vi "environment_get.vi"(0 "reference":refnum<class "OSA.lvclass">, 3 "read defaultValues":bool, 5 "error in (no error)":errorcluster, 9 "parameter":T1(ring)) -> (8 "update temp":bool, 10 "update pressure":bool, 12 "update humidity":bool, 14 "duplicate reference":refnum<class "OSA.lvclass">, 15 "temp (degree C)":sgl format="%.2f", 16 "rel humidity (%)":sgl, 17 "pressure (hPa)":sgl format="%.2f", 19 "error out":errorcluster)   [LabVIEW 2010, in "OSA.lvclass"]
doc: "Interferometer environment."
uses:
  OSA.lvclass
  FTSLib.dll
panel:
  out "par option":i32 format="%b"
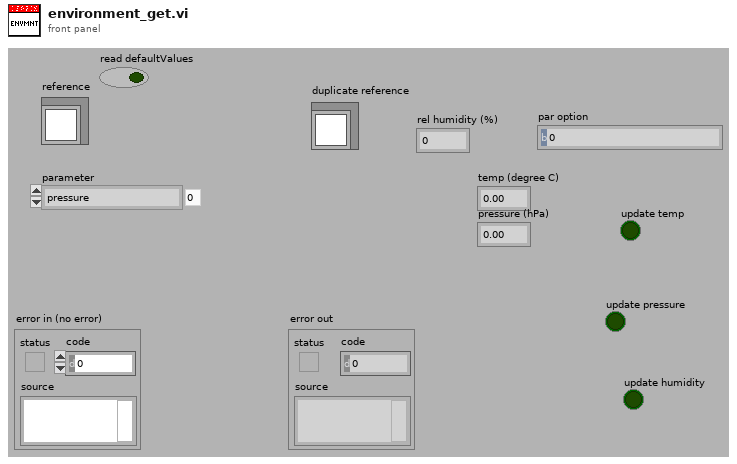
[diagram p1: front panel]
types:
  T1 = enum16{"pressure", "temperature", "humidity", "all"}
  T2 = typedef "OSA.lvclass/ObjectAttributes.ctl" = cluster{"Stop":bool, "dataType":T3, "spectrometerIdx":u16, "buffer size interferogram":i32, "interferogram":cluster{"new":bool, "plot_x_ min":sgl, "plot_x_max":sgl, "plot_y_min":sgl, "plot_y_max":sgl, "Graph Intrfrgrm":T4, "timeStamp":u32, "signal (%)":dbl, "traces":cluster{"idx":u32, "broadBand":bool, "monoChromatic":bool, "peakToPeakSignal":dbl, "peakToPeakPos":dbl}[], "traces idx last":i32, "contrast (%)":dbl}, "spectrum":cluster{"new":bool, "plot_x_min":sgl, "plot_x_max":sgl, "plot_unit_x":T5, "plot_unit_y":T6, "plot_y_min":sgl, "plot_y_max":sgl, "Graph Spectrum":T4, "timeStamp":u32, "X_VAL_OPTIONS":enum16{"MIN_MAX", "ARRAY"}, "traces":cluster{"idx":u32}[], "traces idx last":i32}, "Thorlabs_OSA_64.lvclass:queue_action.ctlqueue ref":refnum<queue>, "action":T7, "plot zoom step":dbl, "buffer semaphore":T8, "acq stopped":bool, "dataType active":T3, "temperature (degr C)":sgl, "pressure (hPa)":sgl, "rel humidity (%)":sgl, "settings":cluster{"resolution":u16, "sensitivity":u16, "Average":bool, "average nr":u32, "apodisation":T9, "acq delay (ms)":u32, "airMesure":T10, "wmtr on":bool, "intfgrm_smooth_width":u16, "intfgrm_smooth_nrOfPasses":u16, "intfgrm_smooth":T11, "phaseCorrection":T12, "zeroFill":u8, "spectr_smooth":T11, "spectr_smooth_width":u16, "spectr_smooth_nrOfPasses":u16, "resolution (/cm)":sgl, "REF wavelength, (nm)":dbl, "gain_idx":u16, "gainAuto":bool, "gain_relative":dbl, "PD sensitivity mode":T13, "PD senseMode implemented":bool, "SensorTemperature implemented":bool, "SensorPressure implemented":bool, "SensorHumidity implemented":bool, "attenuationAuto":bool, "attenuationOnOff":bool, "attenuationAvailable":bool, "offsetAvailable":bool, "offset":i32, "offset max":u16, "contrastAvailable":bool}, "peaks position":sgl[], "peaks width":sgl[], "peaks height":sgl[], "peaks max nr":u32, "peaks latest nr":i32, "peaks new":bool, "power":dbl, "power new":bool, "path":string, "wavelength (WNr)":dbl, "wavelength new":bool, "buffer size spectrum":i32, "status":string, "vi reference":refnum<vi>, "funcPointer":u64, "libraryPointer":u64, "singleAcquisition":bool, "coherenceLength (cm)":dbl, "coherenceLength new":bool, "spectrometer model":string, "spectrometer serial nr":string, "peaks thld left":sgl[], "peaks thld right":sgl[], "coherenceLength error (cm)":dbl, "ADC bits":u16, "peaks position centroid":sgl[], "peaks height centroid":sgl[], "OSA series":T14, "channel index spectrum":u16, "spectrometer rangeLow, (/cm)":dbl, "spectrometer rangeHigh, (/cm)":dbl, "channel index interferogram":u16, "virtualSource":bool, "sweep restart":bool}
  T3 = typedef "OSA.lvclass/acq_dataType.ctl" = enum16{"none", "interferogram", "spectrum"}
  T4 = typedef "OSA.lvclass/graph_intensity.ctl" = refnum<vi>
  T5 = typedef "OSA.lvclass/spectrum_x_unit.ctl" = enum16{"wavenr/cm", "THz", "eV", "nm_air", "nm_vac"}
  T6 = typedef "OSA.lvclass/y_unit.ctl" = enum16{"ADC counts", "dBm pwr absolute", "dBm pwr density", "mW pwr absolute", "mW pwr density"}
  T7 = typedef "OSA.lvclass/queue_action.ctl" = enum16{"none", "stop", "GUI_plotInterferogram", "GUI_plotSpectrum", "GUI_plotInterferogramRescale", "GUI_plotSpectrumRescale", "GUI_plotInterferogramReset", "GUI_plotSpectrumReset", "GUI_plotInterferogramAutoScaleY", "GUI_plotSpectrumAutoScaleY", "GUI_plotInterferogramZoomOut", "GUI_plotSpectrumZoomOut", "GUI_plotInterferogramPane", "GUI_plotSpectrumPane", "GUI_plotInterferogramZoomMouse", "GUI_plotSpectrumZoomMouse", "GUI_spectrumChannelType", "GUI_channel", "ENVIRONMENT temperature", "ENVIRONMENT pressure", "MODE_resolution set", "MODE_resolution get", "MODE_sensitivity set", "MODE_sensitivity get", "MODE_PDTemperature set", "MODE_PDTemperature get", "REBOOT/RESET firmware", "ACQASYNC_acquireSingleSpectrum", "ACQASYNC_continuous start", "ACQASYNC_continuous stop\n", "ACQASYNC_get last interferogram", "ACQASYNC_get last spectrum", "ACQASYNC_get last waveNr", "ACQOPT_interferogram smoothing set", "ACQOPT_interferogram smoothing get", "ACQOPT_spectrum smoothing set", "ACQOPT_spectrum smoothing get", "ACQOPT_apodisation type set", "ACQOPT_apodisation type get", "ACQOPT_phase correction type set", "ACQOPT_phase correction type get", "ACQOPT_acqIntervall_set", "ACQOPT_acqIntervall_get", "ACQOPT_average spectrum set", "ACQOPT_average spectrum get", "ACQOPT_rolling average set", "ACQOPT_rolling average get", "ACQOPT_zero fill factor set", "ACQOPT_zero fill factor get", "ACQOPT_cycle counting set", "ACQOPT_cycle counting get", "ACQOPT_air measure option set", "ACQOPT_air measure option get", "ACQOPT_gainLevel auto get", "ACQOPT_gainLevel auto set", "ACQOPT_gainLevel get", "ACQOPT_gainLevel set", "ACQOPT_offset set", "ACQOPT_attenuator_auto_set", "ACQOPT_attenuator_set", "ACQOPT_getAll", "INSTRUMENT_PROPERTY_range_WaveNr_min", "INSTRUMENT_PROPERTY_range_WaveNr_max", "INSTRUMENT_PROPERTY_reference_wavelength_cm^-1", "INSTRUMENT_PROPERTY_samplesPerRefPeriod", "INSTRUMENT_PROPERTY_resolution_waveNrPercm", "INSTRUMENT_PROPERTY_availableGainLevels", "INSTRUMENT_PROPERTY_status", "CONVERT", "ANALYSE_POWER", "ANALYSE_PEAKS", "ANALYSE_WAVELENGTH", "ANALYSE_SPECTRUM", "ANALYSE_INTERFEROGRAM", "ANALYSE_COHERENCE_LENGTH", "MATH", "MATH_power", "MATH_peaks", "FILE", "miscellaneous"}
  T8 = typedef "Semaphore RefNum" = refnum<k1>
  T9 = typedef "OSA.lvclass/apodisation.ctl" = enum16{"NONE", "NORTON_BEER_WEAK", "NORTON_BEER_MEDIUM", "NORTON_BEER_STRONG", "TRIANGULAR", "COSINE", "HANN", "HAMMING", "BLACKMANHARRIS3", "BLACKMANHARRIS4", "GAUSSIAN"}
  T10 = typedef "OSA.lvclass/airMeasure.ctl" = enum16{"TEMPERATURE", "PRESSURE"}
  T11 = typedef "OSA20X_misc.lvlib/interferogram_smoothing.ctl" = enum16{"NONE", "BINOMIAL", "SAVITSKY_GOLAY", "FOURIER", "MOVING_AVERAGE", "GAUSSIAN"}
  T12 = typedef "OSA.lvclass/phaseCorrection.ctl" = enum16{"NONE", "MERTZ", "FORMAN", "MERTZ_FILE", "FORMAN_FILE", "FUTURE COMP."}
  T13 = typedef "OSA20X_misc.lvlib/PDTemperatureMode.ctl" = enum16{"cool: better sensitivity/noise floor", "warm: extended wl range"}
  T14 = typedef "OSA.lvclass/OSA_series.ctl" = enum16{"OSA200", "OSA300", "UNKNOWN"}
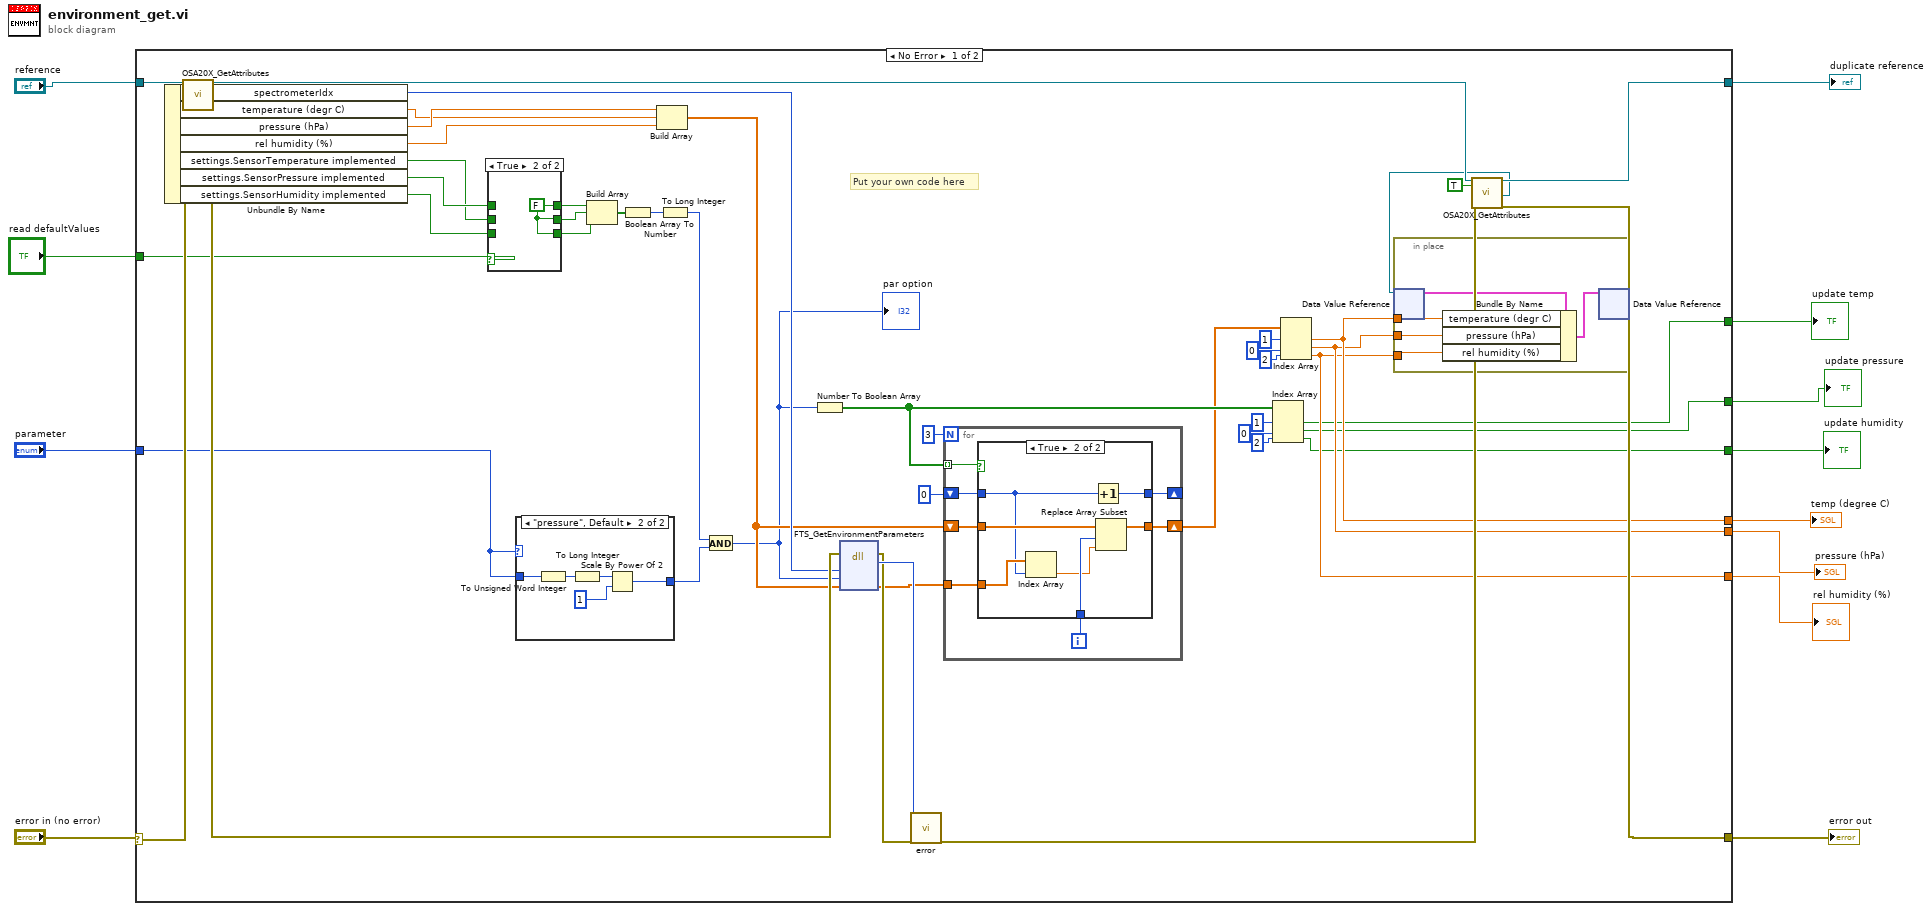
[diagram p0: block diagram]
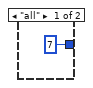
[diagram p4: hidden frame]
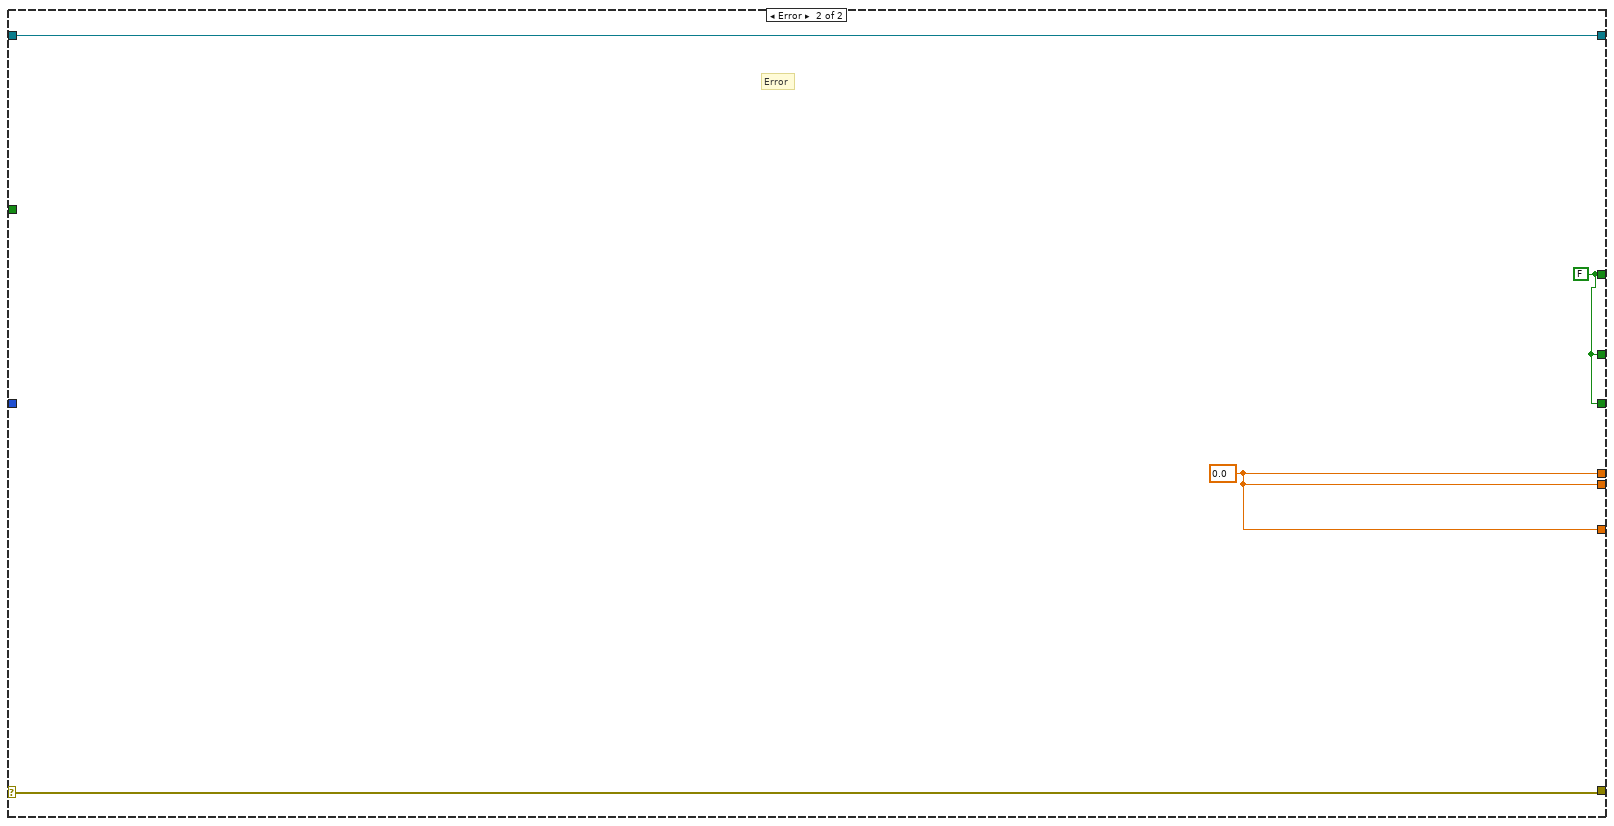
[diagram p5: hidden frame]
diagram:
  n1 = case shown="No Error" "error in (no error)" {
    selector: "error in (no error)" -> [w58 w93]
    tunnel: [w52 w93] -> w12
    tunnel: "reference" -> [w59 w94]
    tunnel: [w54 w94] -> w9
    tunnel: "parameter" -> [w48 _]
    tunnel: [w41 w92] -> w7
    tunnel: [w40 w92] -> w6
    tunnel: [w39 w92] -> w5
    tunnel: [w34 w91] -> w4
    tunnel: [w33 w91] -> w3
    tunnel: [w32 w91] -> w2
    tunnel: "read defaultValues" -> [w22 _]
    frame No Error {
      # "Put your own code here"
      n2 = call "OSA20X_GetAttributes.vi"("reference in"=w59, "error in (no error)"=w58) -> ("reference out"=w55:refnum<class "OSA.lvclass">, "Data"=w50:T2, "error out"=w57:errorcluster)  [unwired: 14 in, 1 out]
      n3 = Unbundle By Name(w50) -> ("spectrometerIdx"=w56:u16, "temperature (degr C)"=w13:sgl, "pressure (hPa)"=w14:sgl, "rel humidity (%)"=w47:sgl, "settings.SensorTemperature implemented"=w15:bool, "settings.SensorPressure implemented"=w16:bool, "settings.SensorHumidity implemented"=w19:bool)
      n4 = case shown="True" w22 {
        tunnel: w16 -> [w62 _]
        tunnel: [w62 w63] -> w21
        tunnel: w15 -> [w61 _]
        tunnel: [w61 w63] -> w20
        tunnel: w19 -> [w60 _]
        tunnel: [w60 w63] -> w18
        frame False {
        }
        frame True {
          w63 = FALSE ("SensorTemperature implemented")
        }
      }
      n5 = case shown="\"pressure\", Default" w48 {
        tunnel: w48 -> [_ w84]
        tunnel: [7 w81] -> w38
        frame "all" {
        }
        frame "pressure", Default {
          n6 = To Unsigned Word Integer(number=w84) -> (unsigned 16bit integer=w85:u16)
          n7 = To Long Integer(number=w85) -> (32bit integer=w83:i32)
          n8 = Scale By Power Of 2(n=w83, x=1 ("32bit integer")) -> (x*2^n=w81:i32)
        }
      }
      n9 = Build Array(w21, w20, w18) -> (w24:bool[])
      n10 = Boolean Array To Number(Boolean array=w24) -> (number=w25:u32)
      n11 = Build Array(w14, w13, w47) -> (w29:sgl[])
      n12 = To Long Integer(number=w25) -> (32bit integer=w23:i32)
      n13 = And(x=w23, y=w38) -> (x .and. y?=w17:i32)
      "par option" <- w17
      n14 = Number To Boolean Array(number=w17) -> (Boolean array=w31:bool[])
      n15 = dll-call lib="FTSLib.dll" fn="FTS_GetEnvironmentParameters"(error in=w57, "spectrIdx"=w56, "parOption"=w17, "par"=w29) -> (error out=w45:errorcluster, "return type"=w46:i32, "par"=w30:sgl[])  [unwired: 4 in, 1 out]
      n16 = call "error.vi"("result code"=w46, "error in (no error)"=w45) -> ("error out"=w53:errorcluster)  [unwired: 15 in, 2 out]
      n17 = for {
        N: 3 -> [_]
        tunnel: w31 -> [w66] mode=indexing
        tunnel: w30 -> [w64]
        shift-right: [w69] -> w27
        shift-left: w29 -> [w70]
        shift-right: [w65] -> _
        shift-left: 0 -> [w67]
        i -> [w68]
        n18 = case shown="True" w66 {
          tunnel: w70 -> [w72 w79]
          tunnel: [w72 w78] -> w69
          tunnel: w68 -> [_ w77]
          tunnel: w67 -> [w71 w74]
          tunnel: [w71 w76] -> w65
          tunnel: w64 -> [_ w75]
          frame False {
          }
          frame True {
            n19 = Index Array(array=w75, index=w74) -> (element=w73:sgl)
            n20 = Increment(x=w74) -> (x+1=w76:i32)
            n21 = Replace Array Subset(array=w79, new element=w73, index=w77) -> (w78:sgl[])
          }
        }
      }
      n22 = Index Array(array=w31, index #1=1 ("index"), index #2=0 ("index"), index #3=2 ("index")) -> (element #1=w34:bool, element #2=w33:bool, element #3=w32:bool)
      n23 = Index Array(array=w27, index #1=1 ("index"), index #2=0 ("index"), index #3=2 ("index")) -> (element #1=w41:sgl, element #2=w40:sgl, element #3=w39:sgl)
      n24 = call "OSA20X_GetAttributes.vi"("reference in"=w55, "OnlyGetDvrReference(False)"=TRUE, "error in (no error)"=w53) -> ("reference out"=w54:refnum<class "OSA.lvclass">, "DataRef"=w49:refnum<data-value>, "error out"=w52:errorcluster)  [unwired: 13 in, 1 out]
      n25 = in-place {
        in-place-border: w41 -> [w88]
        in-place-border: w40 -> [w87]
        in-place-border: w39 -> [w86]
        n26 = in-place-dvr #1(w49) -> (w90:T2)  [unwired: 1 out]
        n27 = Bundle By Name(cluster=w90, "temperature (degr C)"=w88, "pressure (hPa)"=w87, "rel humidity (%)"=w86) -> (w89:T2)
        n28 = in-place-dvr #1(w89) -> ()  [unwired: 2 out]
      }
    }
    frame Error {
      w91 = FALSE
      w92 = sgl 0.0 ("temperature (degr C)")
      # "Error"
    }
  }
  "error out" <- w12
  "duplicate reference" <- w9
  "temp (degree C)" <- w7
  "pressure (hPa)" <- w6
  "rel humidity (%)" <- w5
  "update pressure" <- w3
  "update humidity" <- w2
  "update temp" <- w4
